vi "EstimateAbsoluteOrientation.vi"(7 "Point Set Weights":dbl[](array[numeric]), 8 "error in":errorcluster, 9 "Termination Criterion":refnum<class "Termination Criteria.lvclass">, 10 "Reference Object Point":dbl[][](array[numeric]), 11 "Corresponding Object Points Array":dbl[][][](array[numeric])) -> (0 "error out":errorcluster, 1 "T Vectors":dbl[][](array[numeric]), 2 "R Matricies":dbl[][][](array[numeric]), 3 "Optimized Point Set":T1, 4 "Scale Values":dbl[](array[numeric]))   [LabVIEW 2020, in "g_ar_toolkit.pointset_utils.lvlib" / "Absolute Orientation.lvlib"]
uses:
  Absolute Orientation.lvlib
  Affine Estimation/PointSet.ctl
  g_ar_toolkit.common/Termination Criteria/Termination Criteria.lvclass
  Affine Estimation/Transform.ctl
  <vilib>/Analysis/Matrix/Datatypes/RealMatrix.ctl
  Affine Estimation/SubtractMeanFromPoints.vi
  Affine Estimation/CovarianceofPointSetsA&B.vi
  Affine Estimation/DecomposeCovarianceOfPointSetsA&B.vi
  <vilib>/Analysis/baseanly.llb/A x Vector.vi
  <vilib>/Analysis/baseanly.llb/Mean.vi
  <vilib>/Analysis/baseanly.llb/Mean (DBL).vi
  <vilib>/Analysis/baseanly.llb/A x B.vi
  <vilib>/Analysis/baseanly.llb/Real A x B.vi
  <vilib>/Analysis/baseanly.llb/Determinant.vi
  <vilib>/Analysis/baseanly.llb/Real Determinant.vi
  Affine Estimation/SVDForPointSetCovarainces.vi
  <vilib>/Analysis/_algsub.llb/Matrix Rank.vi
  <vilib>/Analysis/_algsub.llb/Real Matrix Rank.vi
  <vilib>/Analysis/_algsub.llb/Trace.vi
  <vilib>/Analysis/_algsub.llb/Real Matrix Trace.vi
  <vilib>/Utility/error.llb/Error Cluster From Error Code.vi
  <vilib>/Analysis/Matrix/Numeric/Conversions/Array To Matrix - RA2.vi
  <vilib>/Analysis/7linalg.llb/SVD Decomposition.vi
  <vilib>/Analysis/7linalg.llb/Real SVD Decomposition.vi
  <vilib>/Analysis/7linalg.llb/Create Special Matrix.vi
  <vilib>/Analysis/Matrix/Numeric/Multiply/Multiply - RM,R.vi
  <vilib>/ErrorRing/Error Ring.xnode
  Affine Estimation/Affine Estimation.lvlib
  <vilib>/Analysis/Matrix/NI_Matrix.lvlib
  <vilib>/Analysis/NI_AALPro.lvlib
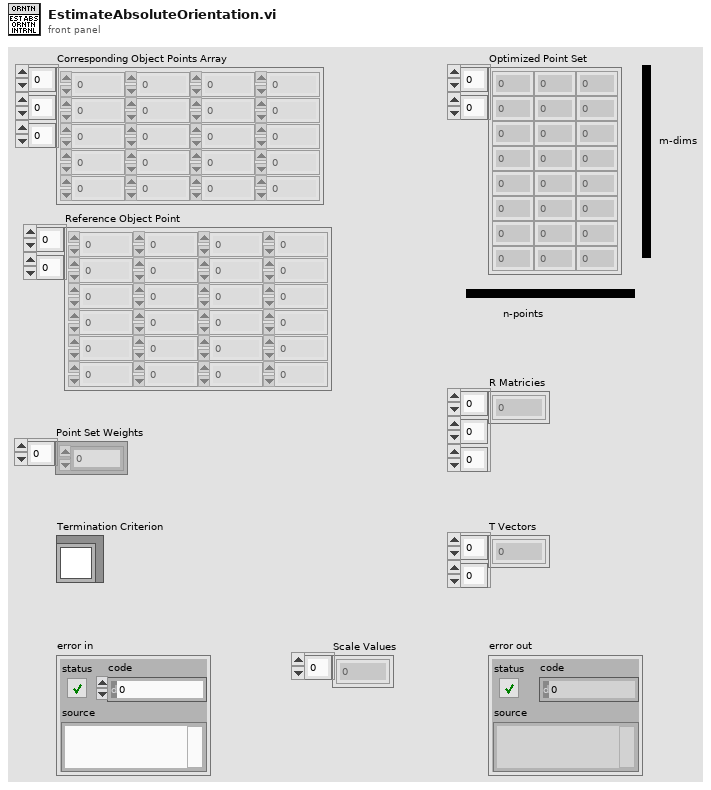
[diagram p1: front panel]
types:
  T1 = typedef "g_ar_toolkit.pointset_utils.lvlib/Affine Estimation.lvlib/PointSet.ctl" = dbl[][]
  T2 = typedef "g_ar_toolkit.pointset_utils.lvlib/Absolute Orientation.lvlib/Transform.ctl" = cluster{"R":T3, "t":dbl[], "c":dbl}
  T3 = typedef "NI_Matrix.lvlib/RealMatrix.ctl" = dbl[][]
  T4 = typedef "g_ar_toolkit.common.lvlib/Termination Criteria.lvclass/Termination Criteria Values.ctl" = cluster{"Epsilon":dbl, "Iterations":i32}
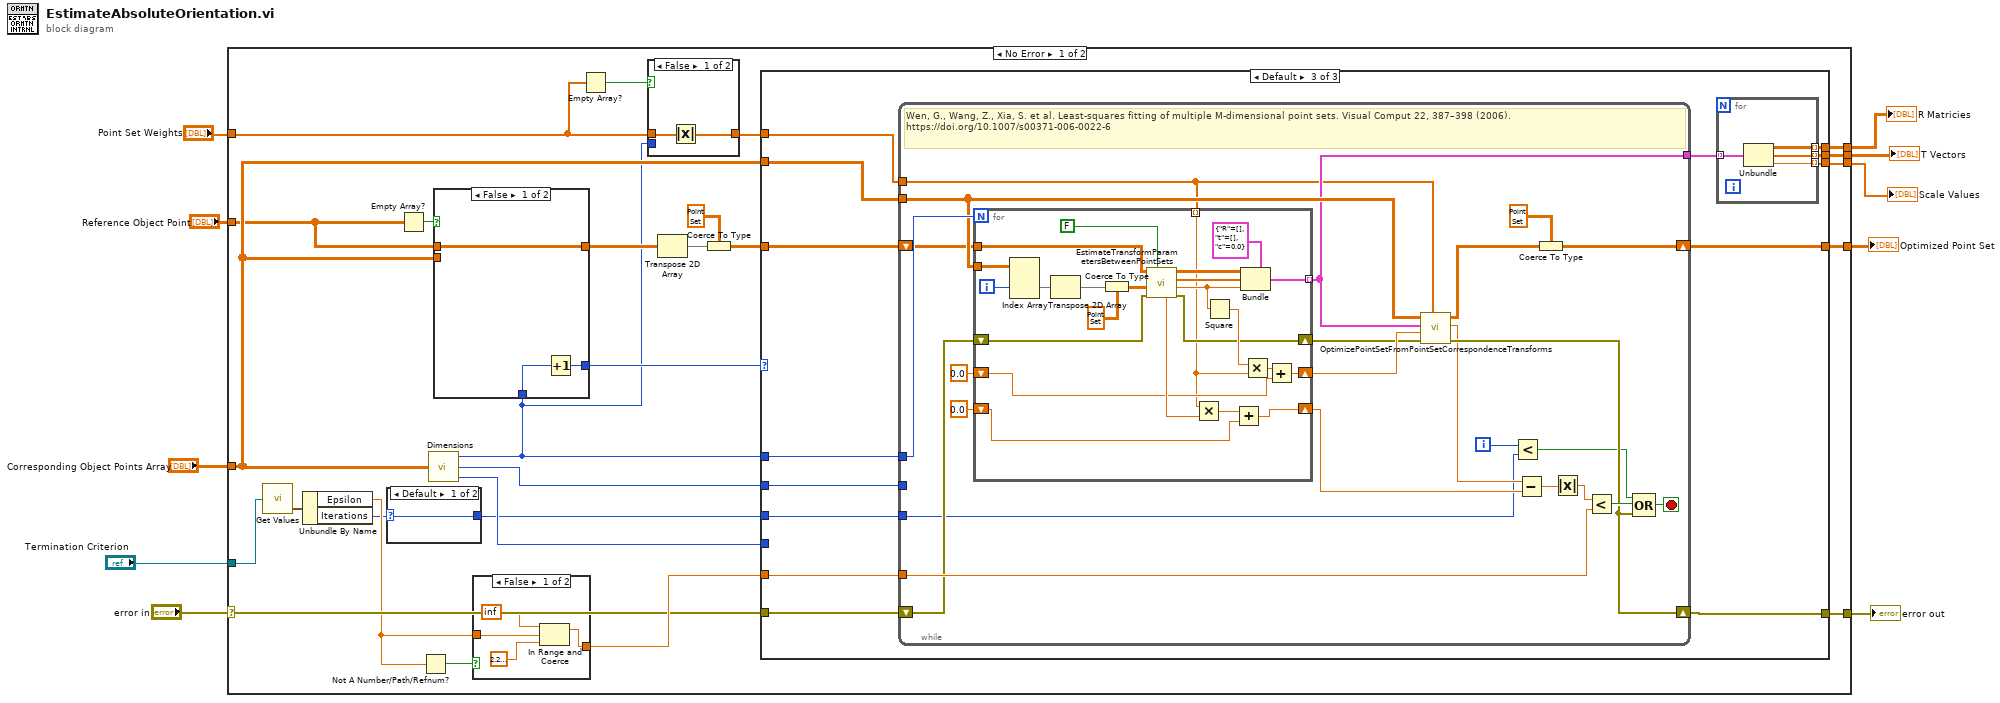
[diagram p0: block diagram]
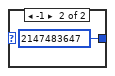
[diagram p2: hidden frame]
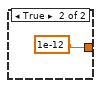
[diagram p3: hidden frame]
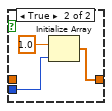
[diagram p4: hidden frame]
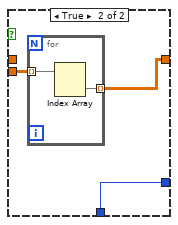
[diagram p5: hidden frame]
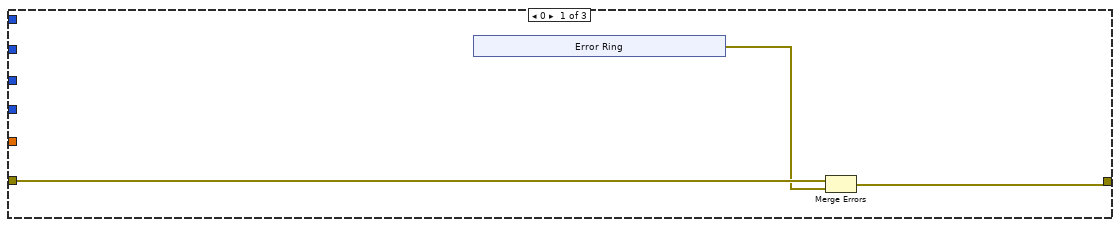
[diagram p6: hidden frame]
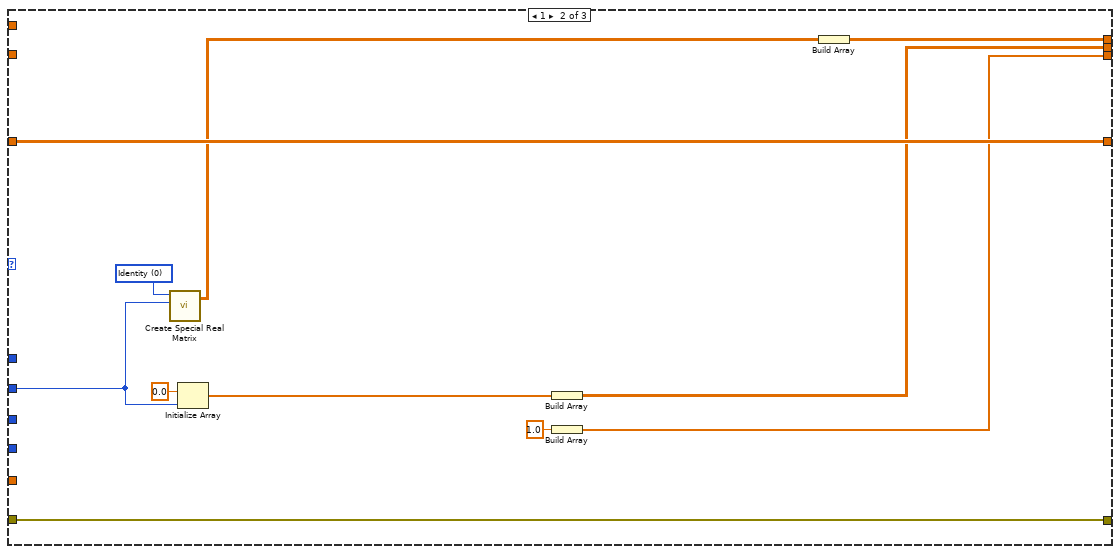
[diagram p7: hidden frame]
diagram:
  n1 = case shown="No Error" "error in" {
    selector: "error in" -> [w25 w143]
    tunnel: "Corresponding Object Points Array" -> [w36 _]
    tunnel: "Reference Object Point" -> [w33 _]
    tunnel: [w30 _] -> w10
    tunnel: [w29 _] -> w9
    tunnel: [w28 _] -> w8
    tunnel: [w27 _] -> w7
    tunnel: "Termination Criterion" -> [w16 _]
    tunnel: [w24 w143] -> w4
    tunnel: "Point Set Weights" -> [w20 _]
    frame No Error {
      n2 = call "Get Values.vi"("Termination Criteria in"=w16) -> ("Term Criteria"=w15:T4)
      n3 = Unbundle By Name(w15) -> ("Epsilon"=w13:dbl, "Iterations"=w12:i32)
      n4 = case shown="Default" w12 {
        selector: w12 -> [w38 _]
        tunnel: [w38 2147483647 ("Iterations")] -> w11
        frame Default {
        }
        frame -1 {
        }
      }
      n5 = Empty Array?(array=w33) -> (empty?=w35:bool)
      n6 = Not A Number/Path/Refnum?(number/path/refnum=w13) -> (NaN/Path/Refnum?=w14:bool)
      n7 = call "Dimensions.vi"("Corresponding Object Points Array"=w36) -> ("k point-sets"=w19:i32, "m dimensions"=w18:i32, "n points in a point set"=w17:i32)  [unwired: 1 in]
      n8 = case shown="False" w35 {
        tunnel: w36 -> [_ w55]
        tunnel: [w52 w54] -> w34
        tunnel: w33 -> [w52 _]
        tunnel: w19 -> [w51 w53]
        tunnel: [w50 w53] -> w23
        frame False {
          n9 = Increment(x=w51) -> (x+1=w50:i32)
        }
        frame True {
          n10 = for {
            tunnel: w55 -> [w57] mode=indexing
            tunnel: [w56] -> w54 mode=indexing
            n11 = Index Array(array=w57) -> (element=w56:dbl[])  [unwired: 2 in]
          }
        }
      }
      n12 = case shown="False" w14 {
        tunnel: [w43 1e-12] -> w26
        tunnel: w13 -> [w40 _]
        frame False {
          n13 = In Range and Coerce(upper limit=inf, x=w40, lower limit=2.220446049250313e-16) -> (coerced(x)=w43:dbl)  [unwired: 1 out]
        }
        frame True {
        }
      }
      n14 = Empty Array?(array=w20) -> (empty?=w22:bool)
      n15 = case shown="False" w22 {
        tunnel: [w45 w49] -> w21
        tunnel: w20 -> [w46 _]
        tunnel: w19 -> [_ w47]
        frame False {
          n16 = Absolute Value(x=w46) -> (abs(x)=w45:dbl[])
        }
        frame True {
          n17 = Initialize Array(1.0 ("element"), w47) -> (w49:dbl[])
        }
      }
      n18 = Transpose 2D Array(2D array=w34) -> (transposed array=w31:dbl[][])
      n19 = Coerce To Type(0:w31, 1:T1 [[0.0, 0.0, 4.0], [0.0, 4.0, 0.0], [0.0, 0.0, 0.0]] ("From Point Set")) -> (2:w37:T1)
      n20 = case shown="Default" w23 {
        tunnel: w18 -> [_ w67 w90]
        tunnel: w37 -> [_ w75 w89]
        tunnel: w36 -> [_ _ w88]
        tunnel: w17 -> [_ _ _]
        tunnel: [_ w73 w86] -> w30
        tunnel: [_ w70 w85] -> w29
        tunnel: [_ w68 w84] -> w28
        tunnel: [_ w75 w83] -> w27
        tunnel: w26 -> [_ _ w82]
        tunnel: w25 -> [w60 w76 w81]
        tunnel: [w59 w76 w80] -> w24
        tunnel: w19 -> [_ _ w78]
        tunnel: w21 -> [_ _ w79]
        tunnel: w11 -> [_ _ w77]
        frame 0 {
          n21 = xnode "Error Ring"() -> ("error out"=w58:errorcluster)
          n22 = Merge Errors(w60, w58) -> (w59:errorcluster)
        }
        frame 1 {
          w66 = 0 items=["Identity", "Diagonal", "Toeplitz", "Vandermonde", "Companion", "Hankel", "Hadamard", "Wilkinson", "Hilbert", "Inverse Hilbert", "Rosser", "Pascal"] ("matrix type")
          n23 = call <vilib>:"Create Special Real Matrix.vi"("matrix type"=w66, "matrix size"=w67) -> ("Special Matrix"=w74:T3)  [unwired: 3 in, 1 out]
          n24 = Initialize Array(0.0 ("element"), w67) -> (w71:dbl[])
          n25 = Build Array(w71) -> (w70:dbl[][])
          n26 = Build Array(1.0) -> (w68:dbl[])
          n27 = Build Array(w74) -> (w73:dbl[][][])
        }
        frame Default {
          n28 = while {
            tunnel: w88 -> [w112]
            tunnel: w78 -> [w113]
            tunnel: w90 -> [_]
            shift-right: [w103] -> w83
            shift-left: w89 -> [w110]
            tunnel: w82 -> [w106]
            tunnel: [w101] -> w87
            shift-right: [w97] -> w80
            shift-left: w81 -> [w100]
            tunnel: w79 -> [w96]
            tunnel: w77 -> [w92]
            i -> [w93]
            stop <- w98 stop-if-true
            # "Wen, G., Wang, Z., Xia, S. et al. Least-squares fitting of multiple M-dimensional point sets. Visual Comput 22, 387–398 (2006).\nhttps://doi.org/10.1007/s00371-006-0022-6"
            n29 = for {
              N: w113 -> [_]
              tunnel: w112 -> [w138]
              tunnel: w110 -> [w124]
              tunnel: [w132] -> w101 mode=indexing
              shift-right: [w130] -> w94
              shift-left: 0.0 ("Minimum Mean Square Error") -> [w129]
              shift-right: [w126] -> w105
              shift-left: 0.0 -> [w125]
              shift-right: [w119] -> w99
              shift-left: w100 -> [w120]
              tunnel: w96 -> [w115] mode=indexing
              i -> [w137]
              n30 = Index Array(array=w138, index (dim 1)=w137) -> (element=w136:dbl[][])  [unwired: 2 in]
              n31 = Transpose 2D Array(2D array=w136) -> (transposed array=w122:dbl[][])
              n32 = Coerce To Type(0:w122, 1:T1 [[0.0, 0.0, 4.0], [0.0, 4.0, 0.0], [0.0, 0.0, 0.0]] ("From Point Set")) -> (2:w121:T1)
              n33 = call "EstimateTransformParametersBetweenPointSets.vi"("Fix Scale at 1.0?"=FALSE, "error in"=w120, "To Point Set"=w121, "From Point Set"=w124) -> ("error out"=w119:errorcluster, "c"=w128:dbl, "t"=w134:dbl[], "R"=w133:T3, "Minimum Mean Square Error"=w131:dbl)  [unwired: 3 in]
              n34 = Multiply(x=w115, y=w131) -> (x*y=w116:dbl)
              n35 = Square(x=w128) -> (x^2=w127:dbl)
              n36 = Add(x=w116, y=w129) -> (x+y=w130:dbl)
              n37 = Bundle(cluster=T2 {"R"=[], "t"=[], "c"=0.0} ("Transform"), "R"=w133, "t"=w134, "c"=w128) -> (w132:T2)
              n38 = Multiply(x=w127, y=w115) -> (x*y=w117:dbl)
              n39 = Add(x=w117, y=w125) -> (x+y=w126:dbl)
            }
            n40 = call "OptimizePointSetFromPointSetCorrespondenceTransforms.vi"("Point Set Weights"=w96, "error in (no error)"=w99, "Sum (v * C^2)"=w105, "Transforms"=w101, "Point Corespondences"=w112) -> ("error out"=w97:errorcluster, "LMS Error"=w95:dbl, "Optimized Points"=w109:dbl[][])  [unwired: 4 in]
            n41 = Less?(x=w93, y=w92) -> (x < y?=w91:bool)
            n42 = Subtract(x=w95, y=w94) -> (x-y=w108:dbl)
            n43 = Coerce To Type(0:w109, 1:T1 [[0.0, 0.0, 4.0], [0.0, 4.0, 0.0], [0.0, 0.0, 0.0]] ("From Point Set")) -> (2:w103:T1)
            n44 = Absolute Value(x=w108) -> (abs(x)=w107:dbl)
            n45 = Less?(x=w107, y=w106) -> (x < y?=w104:bool)
            n46 = Compound Arithmetic op=OR(w91, w104, w97) -> (w98:bool)
          }
          n47 = for {
            tunnel: w87 -> [w142] mode=indexing
            tunnel: [w141] -> w86 mode=indexing
            tunnel: [w140] -> w85 mode=indexing
            tunnel: [w139] -> w84 mode=indexing
            n48 = Unbundle(w142) -> ("R"=w141:T3, "t"=w140:dbl[], "c"=w139:dbl)
          }
        }
      }
    }
    frame Error {
    }
  }
  "error out" <- w4
  "R Matricies" <- w10
  "T Vectors" <- w9
  "Scale Values" <- w8
  "Optimized Point Set" <- w7
